vi "QVA_SetAttributesWhenModified.vi"(0 "QueueIn":refnum<queue>, 2 "SkipAfterTimeout":bool, 3 "VariantData":variant, 5 "ErrorIn":errorcluster) -> (14 "QueueOut":refnum<queue>, 19 "ErrorOut":errorcluster)   [LabVIEW 2016]
doc: "Gibt das Queue Element nach der Bearbeitung zurück. Diese Methode wird nach GettAttributeToModify aufgerufen.\n\nsige / 3.12.13"
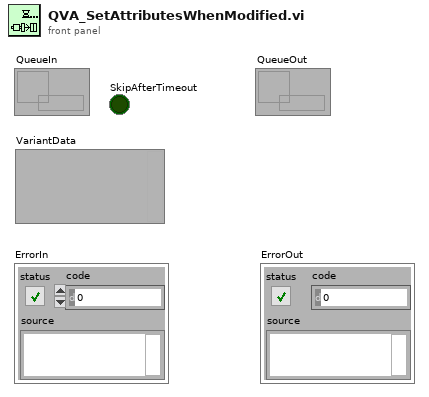
[diagram p1: front panel]
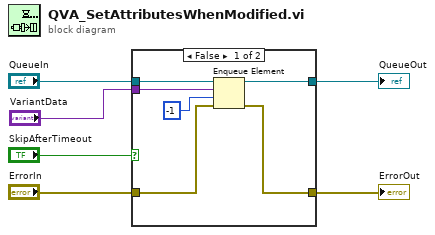
[diagram p0: block diagram]
diagram:
  n1 = case shown="False" "SkipAfterTimeout" {
    tunnel: "ErrorIn" -> [w12 w13]
    tunnel: "QueueIn" -> [w11 w14]
    tunnel: [w10 w14] -> w4
    tunnel: [w9 w13] -> w3
    tunnel: "VariantData" -> [w8 _]
    frame False {
      n2 = Enqueue Element(queue=w11, element=w8, timeout in ms (-1)=-1, error in (no error)=w12) -> (queue out=w10:refnum<queue>, error out=w9:errorcluster)  [unwired: 1 out]
    }
    frame True {
    }
  }
  "QueueOut" <- w4
  "ErrorOut" <- w3
